vi "Meas_Sweep.vi"(0 "SPU":refnum<k24>, 1 "Flag_215":bool, 2 "MPM":refnum<k24>[](array[refnum]), 3 "Data_struct":refnum<k24>[](array[refnum]), 4 "TSL":refnum<k24>, 5 "错误输入（无错误）":errorcluster, 6 "chk2scan":bool, 7 "PDLSTS":refnum<k24>, 8 "Flag_213":bool, 9 "PCU":refnum<k24>, 11 "Meas_monitor_struct":refnum<k24>[](array[refnum]), 12 "Meas_rang":i32[](array[numeric])) -> (19 "错误输出":errorcluster)   [LabVIEW 2017]
uses:
  D:/test/PDLSTS/LV_PDL_Sample/DLL/InstrumentDLL.dll
  DLL/InstrumentDLL.dll
  D:/test/PDLSTS/LV_PDL_Sample/DLL/STSProcess.dll
  DLL/STSProcess.dll
panel:
  in  "sweepcounter":i32
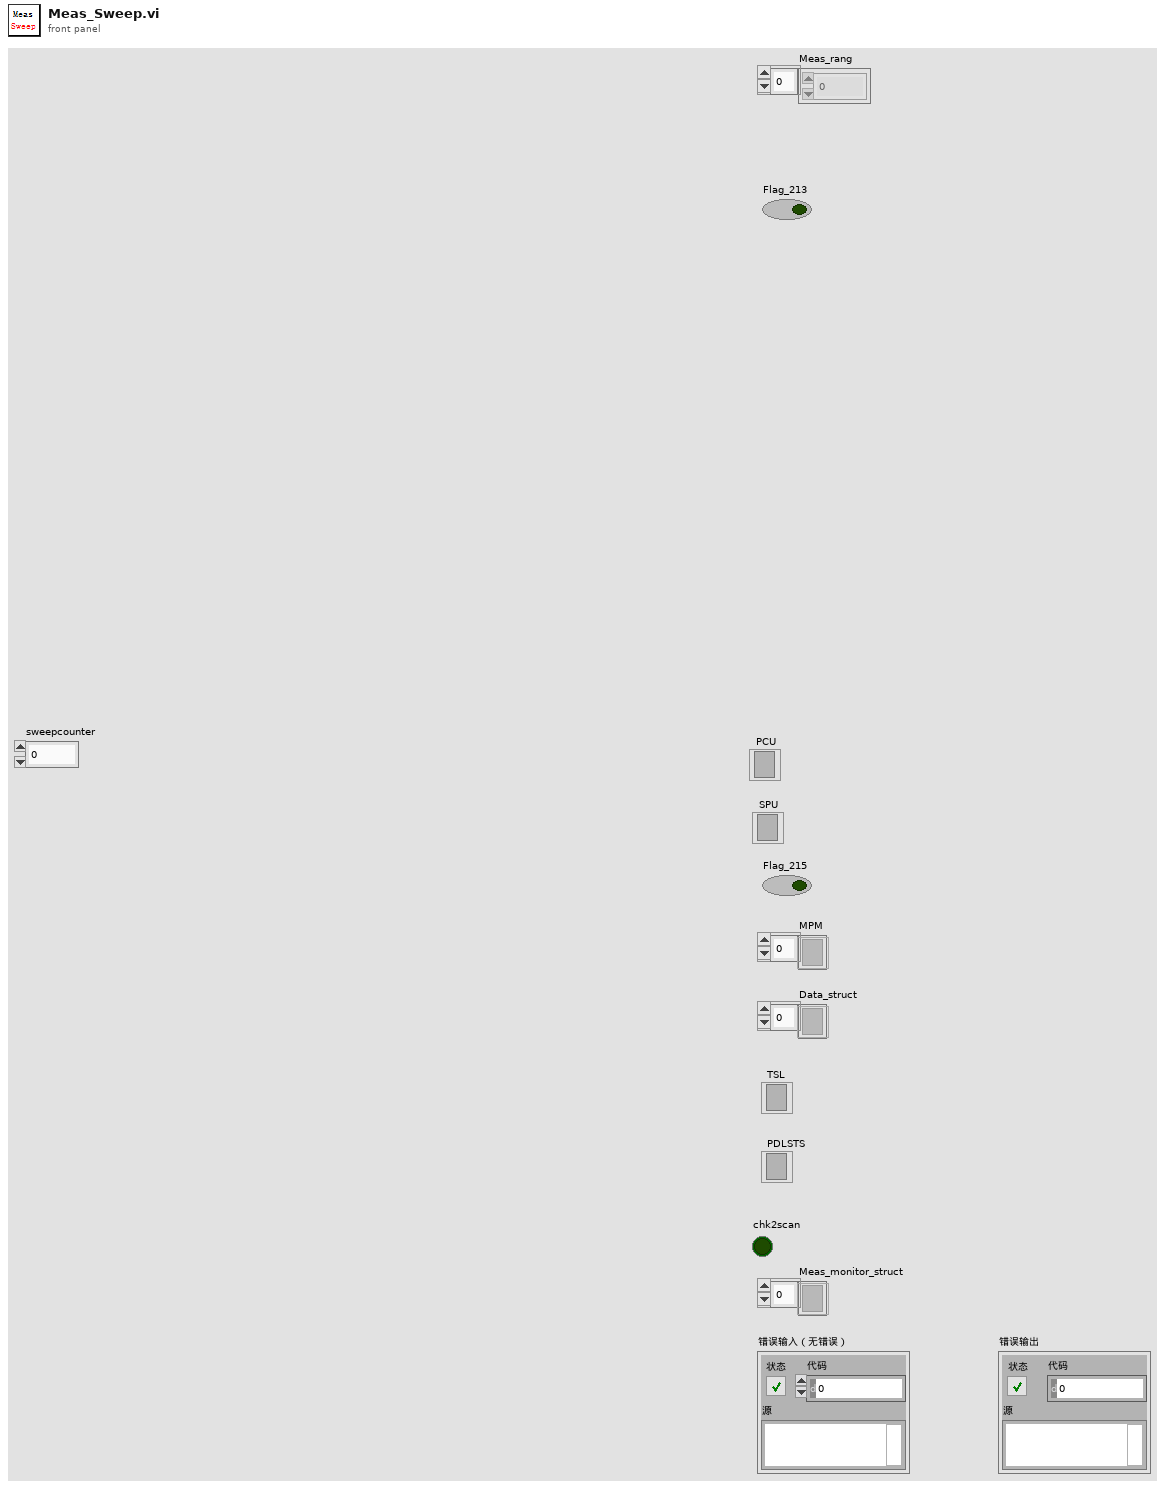
[diagram p1: front panel]
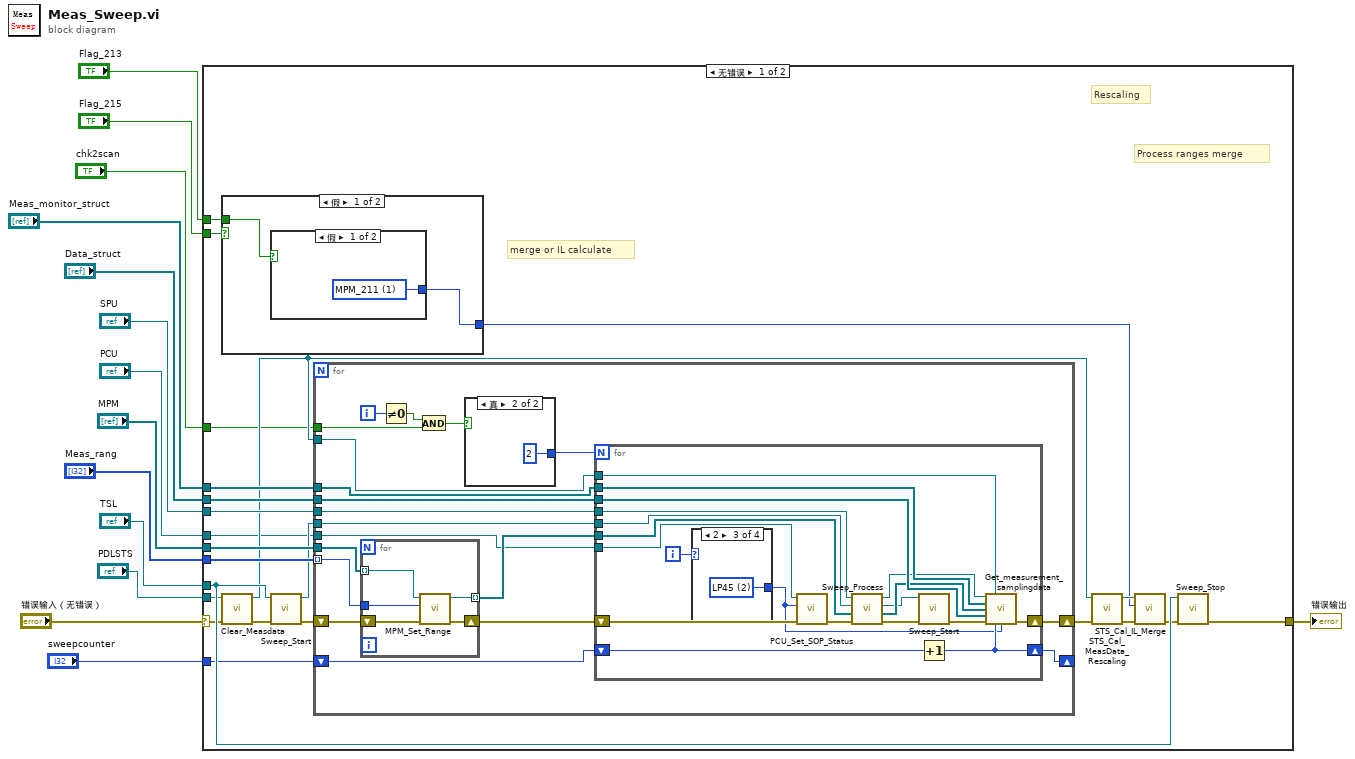
[diagram p0: block diagram]
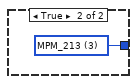
[diagram p2: hidden frame]
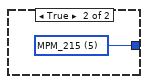
[diagram p3: hidden frame]
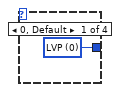
[diagram p4: hidden frame]
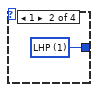
[diagram p5: hidden frame]
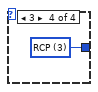
[diagram p6: hidden frame]
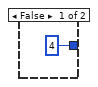
[diagram p7: hidden frame]
diagram:
  n1 = case shown="无错误" "错误输入（无错误）" {
    selector: "错误输入（无错误）" -> [w19 w92]
    tunnel: [w37 w92] -> w14
    tunnel: "Flag_213" -> [w36 _]
    tunnel: "Flag_215" -> [w35 _]
    tunnel: "MPM" -> [w34 _]
    tunnel: "Data_struct" -> [w33 _]
    tunnel: "Meas_monitor_struct" -> [w32 _]
    tunnel: "SPU" -> [w31 _]
    tunnel: "PDLSTS" -> [w21 _]
    tunnel: "Meas_rang" -> [w30 _]
    tunnel: "TSL" -> [w29 _]
    tunnel: "chk2scan" -> [w17 _]
    tunnel: "PCU" -> [w16 _]
    tunnel: "sweepcounter" -> [w15 _]
    frame No Error {
      # "Rescaling"
      # "Process ranges merge"
      # "merge or IL calculate"
      n2 = case shown="假" w35 {
        tunnel: [w39 w42] -> w23
        tunnel: w36 -> [w38 _]
        frame False {
          n3 = case shown="假" w38 {
            tunnel: [w40 w41] -> w39
            frame False {
              w40 = 1 items=["MPM_10"=0, "MPM_211"=1, "MPM_212"=2, "MPM_213"=3, "MPM_215"=5] ("type")
            }
            frame True {
              w41 = 3 items=["MPM_10"=0, "MPM_211"=1, "MPM_212"=2, "MPM_213"=3, "MPM_215"=5] ("type")
            }
          }
        }
        frame True {
          w42 = 5 items=["MPM_10"=0, "MPM_211"=1, "MPM_212"=2, "MPM_213"=3, "MPM_215"=5] ("type")
        }
      }
      n4 = call "Clear_Measdata.vi"("error in (no error)"=w19, ".NET Reference in"=w21) -> ("error out"=w18:errorcluster, "Reference out"=w20:refnum<k24>)  [unwired: 8 in]
      n5 = call "Sweep_Start.vi"("error in (no error)"=w18, ".NET Reference in"=w29) -> ("error out"=w28:errorcluster, "Reference out"=w27:refnum<k24>)  [unwired: 8 in]
      n6 = for {
        tunnel: w30 -> [w60] mode=indexing
        tunnel: w34 -> [w53]
        tunnel: w27 -> [w58]
        tunnel: w31 -> [w54]
        tunnel: w20 -> [w57]
        tunnel: w32 -> [w56]
        tunnel: w33 -> [w55]
        shift-right: [w52] -> w22
        shift-left: w28 -> [w61]
        tunnel: w17 -> [w49]
        tunnel: w16 -> [w46]
        shift-right: [w44] -> _
        shift-left: w15 -> [w43]
        i -> [w45]
        n7 = for {
          tunnel: w53 -> [w91] mode=indexing
          tunnel: w60 -> [w88]
          shift-right: [w89] -> w59
          shift-left: w61 -> [w90]
          tunnel: [w87] -> w51 mode=indexing
          n8 = call "MPM_Set_Range.vi"("error in (no error)"=w90, "Range All"=w88, ".NET Reference in"=w91) -> ("error out"=w89:errorcluster, "Reference out"=w87:refnum<k24>)  [unwired: 7 in]
        }
        n9 = Not Equal To 0?(x=w45) -> (x != 0?=w50:bool)
        n10 = And(x=w50, y=w49) -> (x .and. y?=w48:bool)
        n11 = case shown="真" w48 {
          tunnel: [4 2] -> w47
          frame False {
          }
          frame True {
          }
        }
        n12 = for {
          N: w47 -> [_]
          tunnel: w58 -> [w79]
          tunnel: w57 -> [w78]
          tunnel: w56 -> [w77]
          tunnel: w55 -> [w76]
          tunnel: w54 -> [w75]
          tunnel: w51 -> [w73]
          shift-right: [w74] -> w52
          shift-left: w59 -> [w67]
          tunnel: w46 -> [w65]
          shift-right: [w63] -> w44
          shift-left: w43 -> [w64]
          i -> [w68]
          n13 = case shown="2" w68 {
            tunnel: [w81 w82 w83 w84] -> w62
            frame 0, Default {
              w81 = 0 items=["LVP", "LHP", "LP45", "RCP", "LN45", "LCP"] ("status")
            }
            frame 1 {
              w82 = 1 items=["LVP", "LHP", "LP45", "RCP", "LN45", "LCP"] ("status")
            }
            frame 2 {
              w83 = 2 items=["LVP", "LHP", "LP45", "RCP", "LN45", "LCP"] ("status")
            }
            frame 3 {
              w84 = 3 items=["LVP", "LHP", "LP45", "RCP", "LN45", "LCP"] ("status")
            }
          }
          n14 = call "PCU_Set_SOP_Status.vi"("error in (no error)"=w67, "status"=w62, ".NET Reference in"=w65) -> ("error out"=w66:errorcluster)  [unwired: 7 in, 1 out]
          n15 = call "Sweep_Process.vi"("错误输入（无错误）"=w66, "MPM"=w73, "TSL"=w79, "SPU"=w75) -> ("error out"=w80:errorcluster, "MPM out"=w72:refnum<k24>[], "TSL out"=w71:refnum<k24>, "SPU out"=w70:refnum<k24>)  [unwired: 4 in]
          n16 = call "Sweep_Start.vi"("error in (no error)"=w80, ".NET Reference in"=w71) -> ("error out"=w69:errorcluster)  [unwired: 8 in, 1 out]
          n17 = Increment(x=w64) -> (x+1=w63:i32)
          n18 = call "Get_measurement_samplingdata.vi"("SPU"=w70, "STSProcess.PDLSTS"=w78, "Meas_monitor_struct"=w77, "MPM"=w72, "Data_struct"=w76, "错误输入（无错误）"=w69, "SweepCount"=w63, "SOP"=w62) -> ("error out"=w74:errorcluster)  [unwired: 7 in]
        }
      }
      n19 = call "STS_Cal_MeasData_Rescaling.vi"("错误输入（无错误）"=w22, ".NET引用句柄输入"=w20) -> ("error out"=w24:errorcluster, "引用输出"=w25:refnum<k24>)  [unwired: 8 in]
      n20 = call "STS_Cal_IL_Merge.vi"("错误输入（无错误）"=w24, "type"=w23, ".NET引用句柄输入"=w25) -> ("error out"=w26:errorcluster)  [unwired: 7 in, 1 out]
      n21 = call "Sweep_Stop.vi"("error in (no error)"=w26, ".NET Reference in"=w29) -> ("error out"=w37:errorcluster)  [unwired: 8 in, 1 out]
    }
    frame Error {
    }
  }
  "错误输出" <- w14
